vi "timer-poz.vi"(6 "Czynność":enum16{"reset", "działaj"}(ring), 7 "pauza":bool, 10 "Czas":dbl) -> (3 "czy czas upłynął":bool)   [LabVIEW 2014]
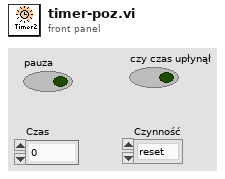
[diagram p1: front panel]
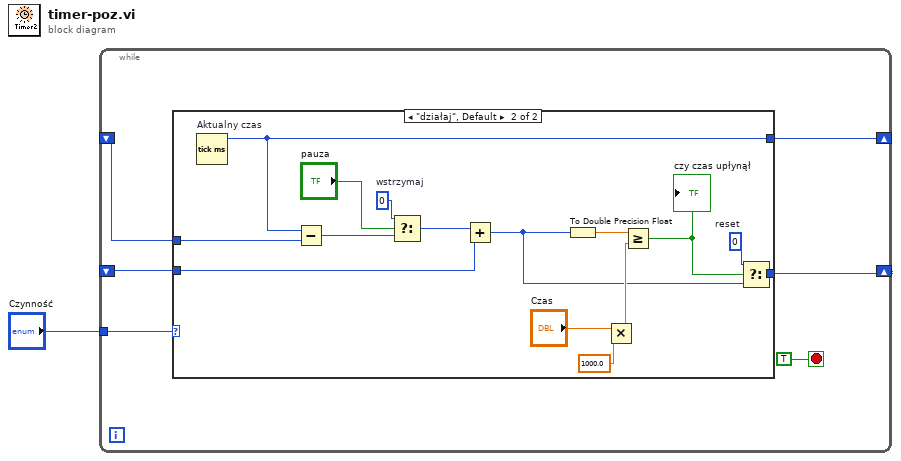
[diagram p0: block diagram]
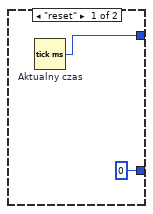
[diagram p2: hidden frame]
diagram:
  n1 = while {
    shift-right: [w4] -> _
    shift-left: _ -> [w3]
    shift-right: [w5] -> _
    shift-left: _ -> [w6]
    tunnel: "Czynność" -> [w2]
    stop <- TRUE stop-if-true
    n2 = case shown="\"działaj\", Default" w2 {
      tunnel: w6 -> [_ w15]
      tunnel: [u32 0 ("reset") w14] -> w5
      tunnel: [w9 w13] -> w4
      tunnel: w3 -> [_ w12]
      frame "reset" {
        n3 = Tick Count (ms) "Aktualny czas"() -> (millisecond timer value=w9:u32)
      }
      frame "działaj", Default {
        w23 = u32 0  # wstrzymaj
        w20 = u32 0  # reset
        n4 = Tick Count (ms) "Aktualny czas"() -> (millisecond timer value=w13:u32)
        n5 = Subtract(x=w13, y=w12) -> (x-y=w22:u32)
        n6 = Select(t=w23, s="pauza", f=w22) -> (s? t:f=w24:u32)
        n7 = Add(x=w24, y=w15) -> (x+y=w11:u32)
        n8 = To Double Precision Float(number=w11) -> (double precision float=w10:dbl)
        n9 = Multiply(x="Czas", y=1000.0) -> (x*y=w19:dbl)
        n10 = Greater Or Equal?(x=w10, y=w19) -> (x >= y?=w21:bool)
        "czy czas upłynął" <- w21
        n11 = Select(t=w20, s=w21, f=w11) -> (s? t:f=w14:u32)
      }
    }
  }
